vi "1feladat.vi"() -> ()   [LabVIEW 2016]
panel:
  out "Numeric 2":dbl
  in  "Numeric":dbl
  out "Boolean 2":bool
  in  "Boolean":bool
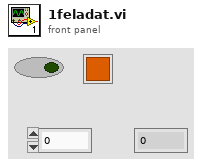
[diagram p1: front panel]
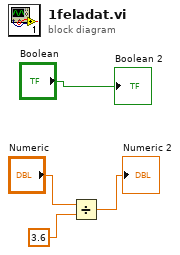
[diagram p0: block diagram]
diagram:
  n1 = Divide(x="Numeric", y=3.6) -> (x/y=→"Numeric 2":dbl)
  "Boolean 2" <- "Boolean"
